vi "New Value Change Subscription.vi"(10 "Ignore Past Updates? (F)":bool, 11 "ValueChangeSubscription In":refnum<class "ValueChangeSubscription.lvclass">) -> (3 "ValueChangeSubscription Out":refnum<class "ValueChangeSubscription.lvclass">)   [LabVIEW 2015, in "Mediator.lvlib" / "ValueChangeSubscription.lvclass"]
uses:
  ValueChangeSubscription.lvclass
  ValueChangeSubscription.lvclass/ValueChangeSubscription.ctl
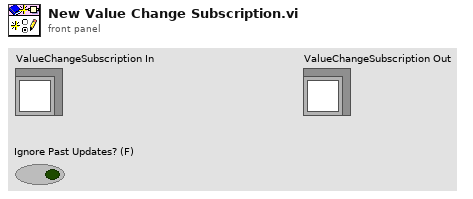
[diagram p1: front panel]
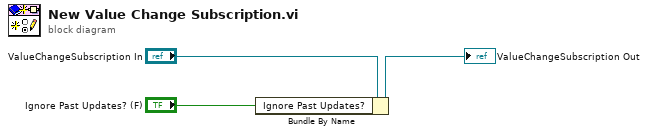
[diagram p0: block diagram]
diagram:
  n1 = Bundle By Name(cluster="ValueChangeSubscription In", "Ignore Past Updates?"="Ignore Past Updates? (F)") -> (→"ValueChangeSubscription Out":refnum<class "ValueChangeSubscription.lvclass">)
